vi "CloseSink.vi"(8 "error in (no error)":errorcluster, 11 "Appender in":refnum<class "Appender.lvclass">) -> (0 "error out":errorcluster, 3 "Appender out":refnum<class "Appender.lvclass">)   [LabVIEW 2026, in "Lumberjack.lvlib" / "Appender.lvclass"]
doc: "Flush and close this appender's sink resource. Called once on actor exit (from Actor Core), including the error-exit path, so buffered data is not lost on shutdown. Abstract: each concrete appender closes its own sink. DD, must override."
uses:
  Appender.lvclass
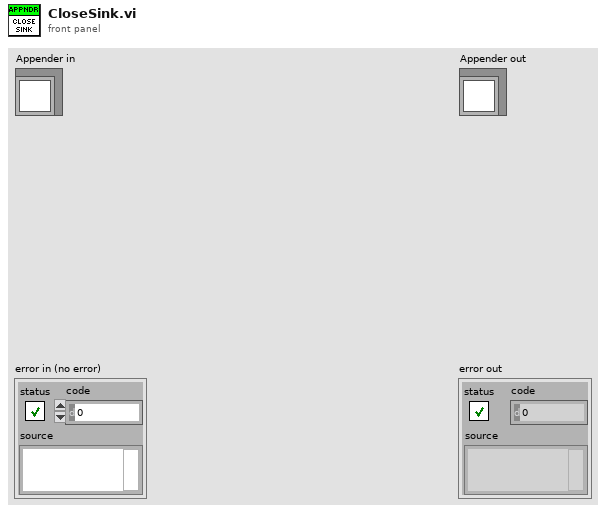
[diagram p1: front panel]
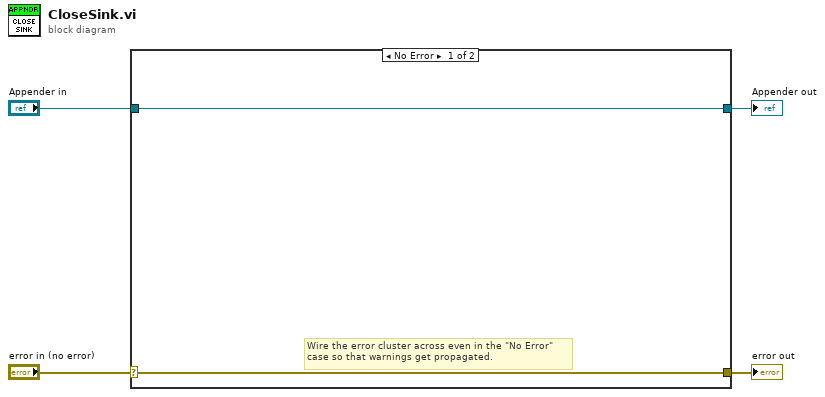
[diagram p0: block diagram]
diagram:
  n1 = case shown="No Error" "error in (no error)" {
    selector: "error in (no error)" -> [w5 w8]
    tunnel: [w5 w8] -> w3
    tunnel: [w6 w7] -> w1
    tunnel: "Appender in" -> [w6 w7]
    frame No Error {
      # "Wire the error cluster across even in the \"No Error\"\ncase so that warnings get propagated."
    }
    frame Error {
    }
  }
  "error out" <- w3
  "Appender out" <- w1
